vi "DataWrite_RTU (SubVI).vi"(2 "Data":dbl, 3 "Address":string="1000", 4 "Select Device":u16) -> (0 "CRC":string, 1 "Write frame":string)   [LabVIEW 2020]
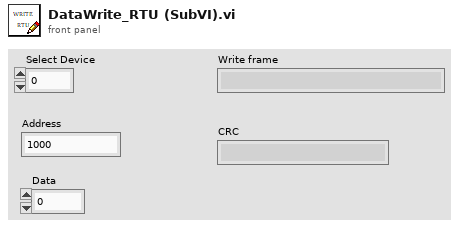
[diagram p1: front panel]
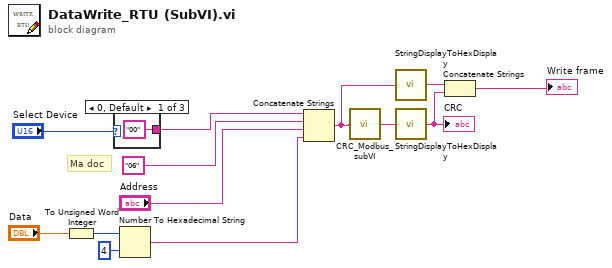
[diagram p0: block diagram]
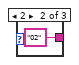
[diagram p2: hidden frame]
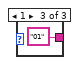
[diagram p3: hidden frame]
diagram:
  # "Ma doc"
  n1 = To Unsigned Word Integer(number="Data") -> (unsigned 16bit integer=w4:u16)
  n2 = case shown="0, Default" "Select Device" {
    tunnel: ["00" ("string") "02" ("string") "01" ("string")] -> w8
    frame 0, Default {
    }
    frame 2 {
    }
    frame 1 {
    }
  }
  n3 = Number To Hexadecimal String(1:i16 4 ("width (-)"), 2:w4) -> (0:w1:string)
  n4 = Concatenate Strings(w8, "06" ("string"), "Address", w1) -> (w9:string)
  n5 = call "CRC_Modbus_subVI.vi"("Before CRC"=w9) -> ("CRC Check"=w13:string)
  n6 = call "StringDisplayToHexDisplay.vi"("Hex Num (Normal Display)"=w9) -> ("Hex Num (Hex Display)"=w12:string)
  n7 = call "StringDisplayToHexDisplay.vi"("Hex Num (Normal Display)"=w13) -> ("Hex Num (Hex Display)"=w10:string)
  "CRC" <- w10
  n8 = Concatenate Strings(w12, w10) -> (→"Write frame":string)
